vi "izolovanje povorke.vi"(11 "Filtered Signal":dynamicdata(waveform)) -> (2 "spektar izolovane povorke":cluster{"f0":dbl, "df":dbl, "magnitude":dbl[]}(graph), 3 "izolovana povorka":waveform(dbl)(graph))   [LabVIEW 2018]
uses:
  <vilib>/Waveform/WDTOps.llb/WDT Get Waveform Subset DBL.vi
  <vilib>/express/express analysis/Spectral/Block/exnSpectralBlock spectral measurements RMS poly.vi
  <vilib>/express/express analysis/Spectral/Block/exnSpectralBlock spectral measurements RMS WFM.vi
  <vilib>/express/express analysis/Spectral/XNode/ExpressSpectralMeasurementsBlockNode.xnode
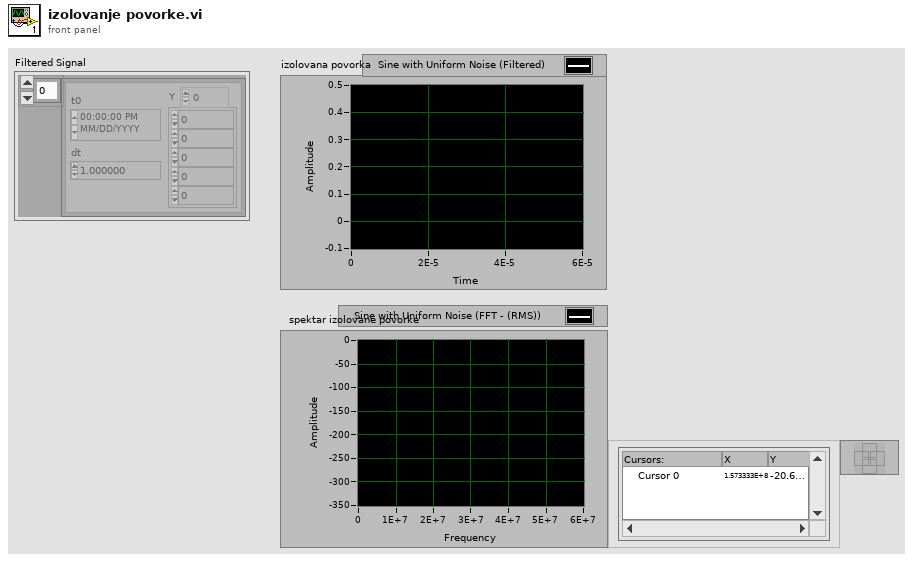
[diagram p1: front panel]
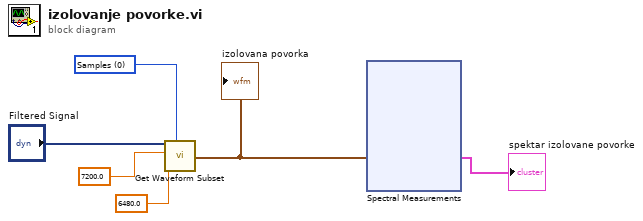
[diagram p0: block diagram]
diagram:
  w3 = u16 0 items=["Samples", "Relative Time"] ("start/duration format")
  n1 = call-poly <vilib>:"Get Waveform Subset.vi"("start/duration format"=w3, "duration"=6480.0, "start samples/time"=7200.0, "waveform in"="Filtered Signal") -> ("waveform out"=w6:waveform(dbl))  [unwired: 2 in, 3 out]
  "izolovana povorka" <- w6
  n2 = xnode "Spectral Measurements"("Signals"=w6) -> ("FFT - (RMS)"=→"spektar izolovane povorke":cluster{"f0":dbl, "df":dbl, "magnitude":dbl[]})  [unwired: 1 in, 2 out]
